vi "Request Data JSON.vi"(8 "error in (no error)":errorcluster, 11 "GetSceneItemTransform in":refnum<class "GetSceneItemTransform.lvclass">) -> (0 "error out":errorcluster, 2 "Request Data JSON":string, 3 "GetSceneItemTransform out":refnum<class "GetSceneItemTransform.lvclass">)   [LabVIEW 2020, in "obs-websocket.lvlib" / "GetSceneItemTransform.lvclass"]
uses:
  GetSceneItemTransform.lvclass
  GetSceneItemTransform.lvclass/GetSceneItemTransform.ctl
  940a11be-9bf9-4a40-915c-8ecb22b27a63.vi
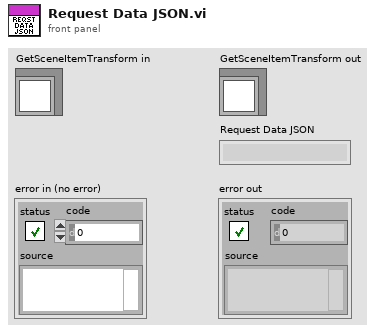
[diagram p1: front panel]
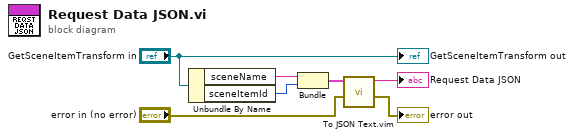
[diagram p0: block diagram]
diagram:
  n1 = Unbundle By Name("GetSceneItemTransform in") -> ("sceneName"=w7:string, "sceneItemId"=w6:i32)
  n2 = Bundle("sceneName"=w7, "sceneItemId"=w6) -> (w5:cluster{"sceneName":string, "sceneItemId":i32})  [unwired: 1 in]
  n3 = call "To JSON Text.vim"("error in (no error)"="error in (no error)", "Anything"=w5) -> ("error out"=→"error out":errorcluster, "<JSON>"=→"Request Data JSON":string)  [unwired: 8 in]
  "GetSceneItemTransform out" <- "GetSceneItemTransform in"
